vi "Exception Handling.vi"(8 "error in (no error)":errorcluster, 9 "Exception Handler Map":T1, 11 "Processing In":refnum<class "Processing.lvclass">) -> (0 "error out":errorcluster, 3 "HTTP Server.lvlib:Processing":refnum<class "Processing.lvclass">)   [LabVIEW 2020, in "HTTP Server.lvlib" / "Server.lvclass"]
uses:
  Server.lvclass
  Server.lvclass/Server.ctl
  Processing Step.ctl
  HTTP Server.lvlib
  Processing/Processing.lvclass
  Exception Handler/Exception Handler.lvclass
  Priority.ctl
  Exception Handler Map.ctl
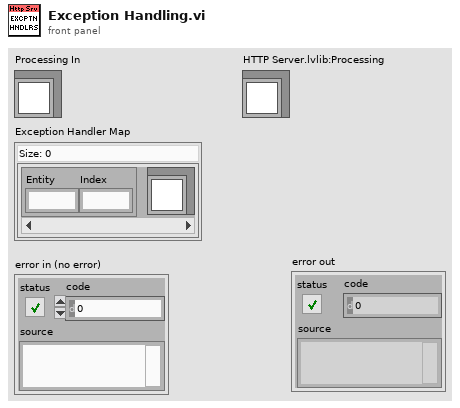
[diagram p1: front panel]
types:
  T1 = typedef "HTTP Server.lvlib/Exception Handler Map.ctl" = map{T2, refnum<class "Exception Handler.lvclass">}
  T2 = typedef "HTTP Server.lvlib/Priority.ctl" = cluster{"Entity":u16, "Index":u16}
  T3 = typedef "HTTP Server.lvlib/Processing Step.ctl" = enum16{"Connection", "Request", "Routing", "Controller Init", "Controller", "Response", "Complete", "Exception"}
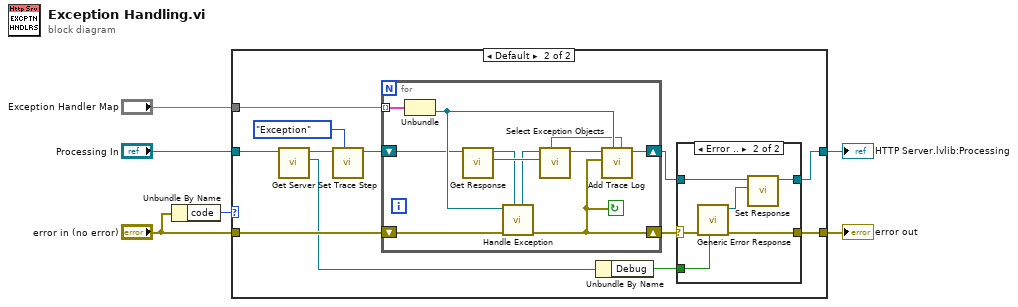
[diagram p0: block diagram]
diagram:
  n1 = Unbundle By Name("error in (no error)") -> ("code"=w1:i32)
  n2 = case shown="Default" w1 {
    tunnel: "Exception Handler Map" -> [_ w20]
    tunnel: "Processing In" -> [w8 w14]
    tunnel: "error in (no error)" -> [w7 w19]
    tunnel: [w7 w18] -> w3
    tunnel: [w8 w10] -> w2
    frame 66 {
      # "Lost connection to client, no sense trying to provide a meaningful response."
    }
    frame Default {
      n3 = call "Get Server.vi"("Processing in"=w14) -> ("Server"=w12:refnum<class "Server.lvclass">, "Processing out"=w13:refnum<class "Processing.lvclass">)  [unwired: 9 in]
      n4 = call "Set Trace Step.vi"("Processing Step"=Processing_Step."Exception", "Processing in"=w13) -> ("Processing out"=w15:refnum<class "Processing.lvclass">)  [unwired: 9 in]
      n5 = for {
        tunnel: w20 -> [w29] mode=indexing
        shift-right: [w27] -> w11
        shift-left: w15 -> [w22]
        shift-right: [w30] -> w17
        shift-left: w19 -> [w28]
        stop <- w30 continue-if-true
        n6 = Unbundle(w29) -> ("Handler"=w26:refnum<class "Exception Handler.lvclass">)  [unwired: 1 out]
        n7 = call "Get Response.vi"("Processing in"=w22) -> ("Response"=w31:refnum<class "Response.lvclass">, "Processing out"=w21:refnum<class "Processing.lvclass">)  [unwired: 9 in]
        n8 = call-dynamic "Handle Exception.vi"("Processing In"=w21, "error in (no error)"=w28, "Exception Handler in"=w26) -> ("error out"=w30:errorcluster, "Processing"=w23:refnum<class "Processing.lvclass">)  [unwired: 7 in]
        n9 = call "Select Exception Objects.vi"("Response"=w31, "Processing"=w23) -> ("Updated Inputs"=w24:refnum<class "Processing.lvclass">, "Trace Message"=w25:string)  [unwired: 8 in]
        n10 = call "Add Trace Log.vi"("Info"=w25, "LabVIEW Object"=w26, "error in (no error)"=w30, "Processing in"=w24) -> ("Processing out"=w27:refnum<class "Processing.lvclass">)  [unwired: 6 in, 1 out]
      }
      n11 = Unbundle By Name(w12) -> ("Debug"=w16:bool)
      n12 = case shown="Error .." w17 {
        selector: w17 -> [w33 w38]
        tunnel: [w33 w39] -> w18
        tunnel: w16 -> [_ w37]
        tunnel: w11 -> [w32 w36]
        tunnel: [w32 w35] -> w10
        frame No Error {
        }
        frame Error {
          n13 = call "Generic Error Response.vi"("Include Message?"=w37, "error in (no error)"=w38) -> ("error out"=w39:errorcluster, "Response out"=w34:refnum<class "Response.lvclass">)  [unwired: 8 in]
          n14 = call "Set Response.vi"("Response"=w34, "Processing in"=w36) -> ("Processing out"=w35:refnum<class "Processing.lvclass">)  [unwired: 9 in]
        }
      }
    }
  }
  "HTTP Server.lvlib:Processing" <- w2
  "error out" <- w3
